vi "Read File - not read spreadsheet.vi"() -> ()   [LabVIEW 2014]
panel:
  out "Array":dbl[][](array[numeric])
  out "number":dbl[][](array[numeric])
  out "subarray":string[][](array[string])
  out "array":string[][](array[string])
  out "text":string
  in  "file path (use dialog)":path
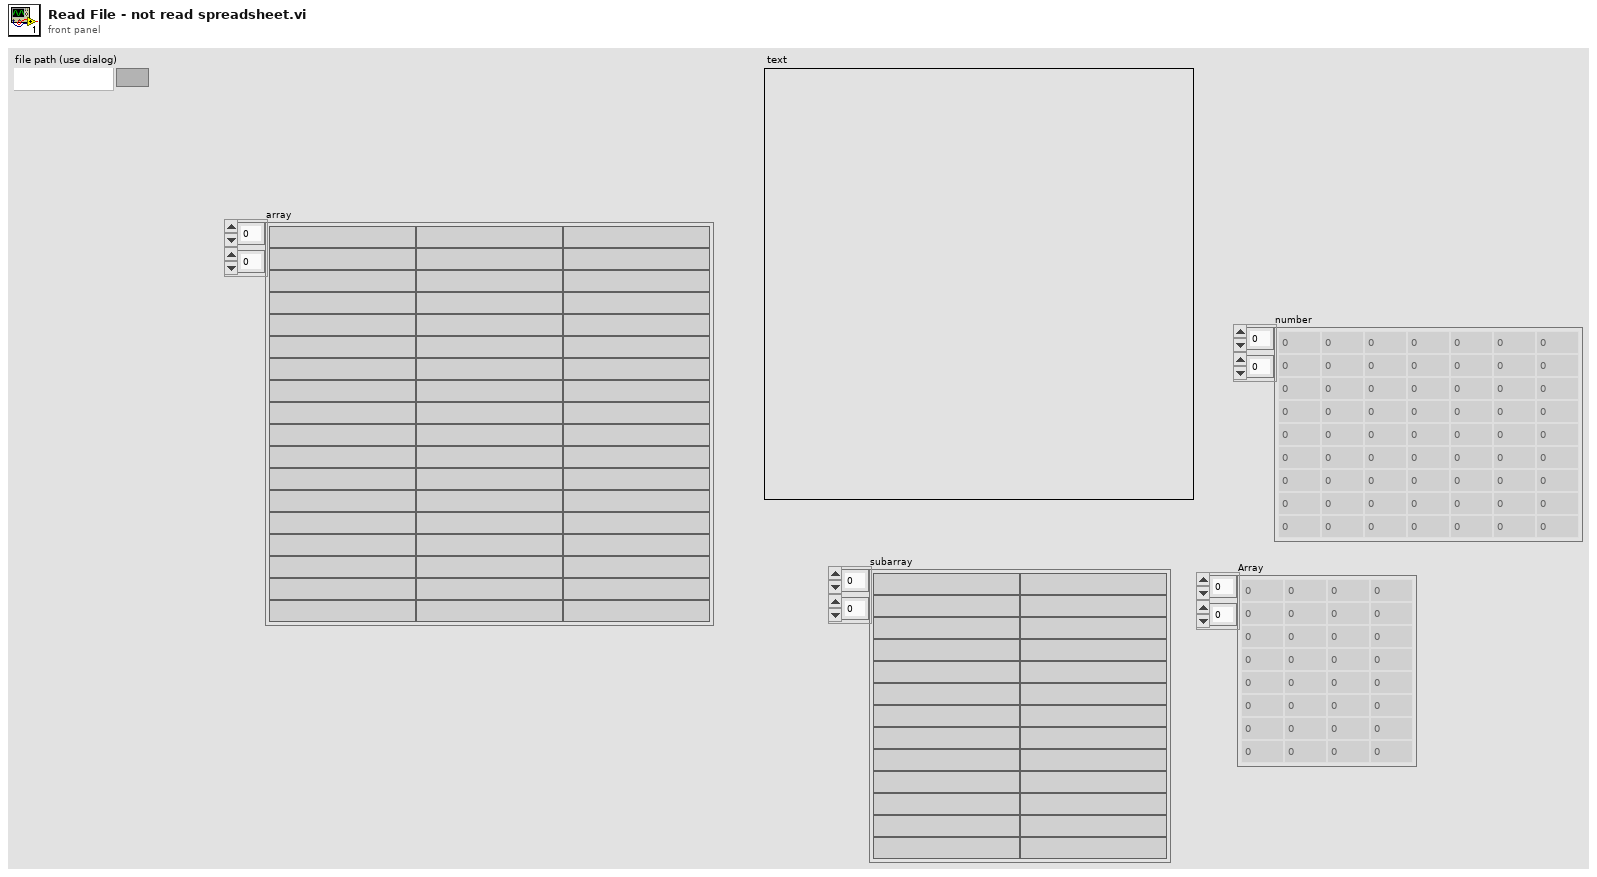
[diagram p1: front panel]
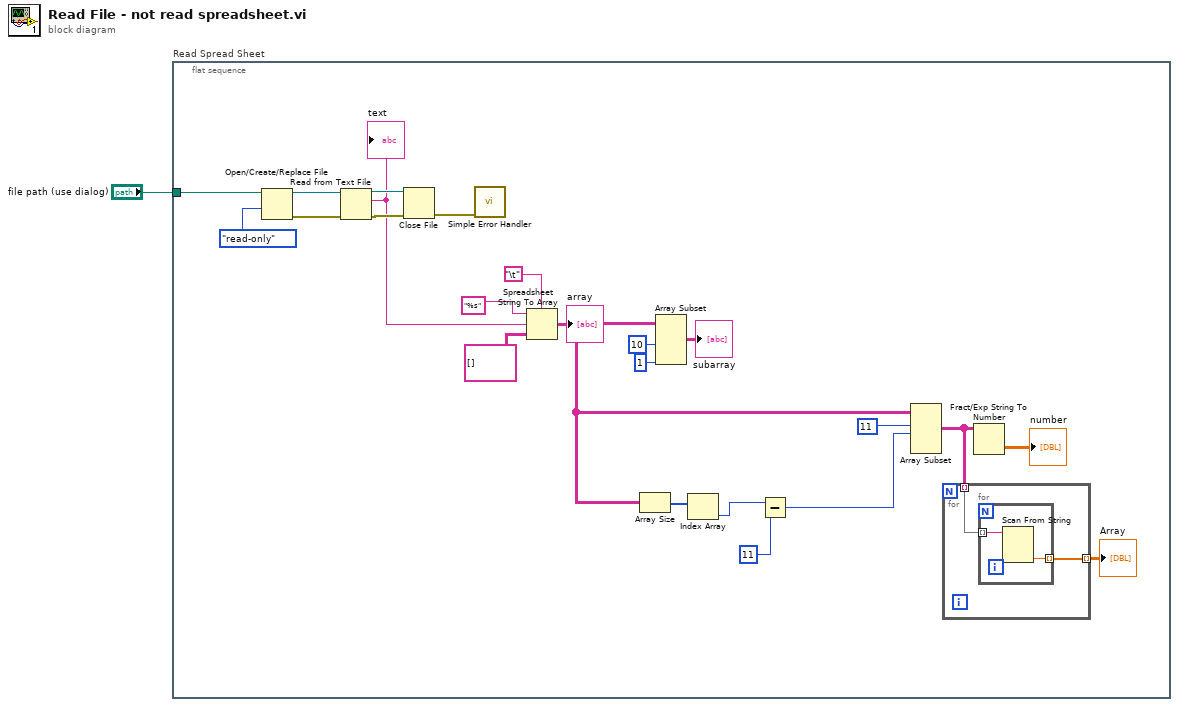
[diagram p0: block diagram]
diagram:
  n1 = flat-sequence "Read Spread Sheet" {
    tunnel: "file path (use dialog)" -> [w24]
    frame #0 {
      n2 = Open/Create/Replace File(file path (use dialog)=w24, access (0:read/write)=enum16{"read/write", "read-only", "write-only"}."read-only") -> (refnum out=w22:refnum<file>, error out=w23:errorcluster)  [unwired: 4 in, 1 out]
      n3 = Read from Text File(file (use dialog)=w22, error in=w23) -> (refnum out=w20:refnum<file>, text=w17:string, error out=w21:errorcluster)  [unwired: 2 in, 1 out]
      "text" <- w17
      n4 = Close File(refnum=w20, error in=w21) -> (error out=w18:errorcluster)  [unwired: 1 out]
      n5 = call <vilib>:"Simple Error Handler.vi"("error in (no error)"=w18) -> ()  [unwired: 4 in, 5 out]
      n6 = Spreadsheet String To Array(delimiter (Tab)="\t", format string="%s", spreadsheet string=w17, array type (2D Dbl)=string[][] []) -> (array=w9:string[][])
      "array" <- w9
      n7 = Array Size(array=w9) -> (size(s)=w8:i32[])
      n8 = Array Subset(array=w9, length (row)=10 ("length"), length (col)=1 ("length")) -> (→"subarray":string[][])  [unwired: 2 in]
      n9 = Index Array(array=w8) -> (element=w7:i32)  [unwired: 1 in]
      n10 = Subtract(x=w7, y=11 ("length")) -> (x-y=w5:i32)
      n11 = Array Subset(array=w9, index (row)=11 ("length"), length (row)=w5) -> (w3:string[][])  [unwired: 2 in]
      n12 = for {
        tunnel: w3 -> [w26] mode=indexing
        tunnel: [w25] -> w2 mode=indexing
        n13 = for {
          tunnel: w26 -> [w28] mode=indexing
          tunnel: [w27] -> w25 mode=indexing
          n14 = Scan From String(input string=w28) -> (output 1=w27:dbl)  [unwired: 4 in, 3 out]
        }
      }
      "Array" <- w2
      n15 = Fract/Exp String To Number(string=w3) -> (number=→"number":dbl[][])  [unwired: 3 in, 1 out]
    }
  }
